vi "UV-VIS SetFastExtTriggerSD.vi"(3 "error in (no error)":errorcluster, 4 "mode":bool, 5 "Control in":refnum<class "CCD_camera.lvclass">) -> (0 "error out":errorcluster, 1 "DLL error code":u32, 2 "Control out":refnum<class "CCD_camera.lvclass">)   [LabVIEW 2018, in "CCD_camera.lvclass"]
doc: "This function will enable fast external triggering. When fast external triggering is enabled the system will NOT wait until a \"Keep Clean\" cycle has been completed before accepting the next trigger. This setting will only have an effect is the trigger mode has been set to External via <B>SetTriggerMode</B>.\n\n<B>Parameter:</B>\nmode - FALSE - Disabled\n TRUE - Enabled\n\n<B>Error code:</B>\nDRV_SUCCESS - Parameters accepted."
uses:
  CCD_camera.lvclass
  C:/Users/Sergey Denisov/Documents/REPS/TRANCON/Classes/Detector/Detector.lvclass
  Detector.lvclass/Detector.ctl
  Detector.lvclass
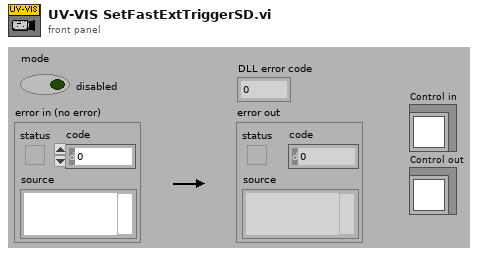
[diagram p1: front panel]
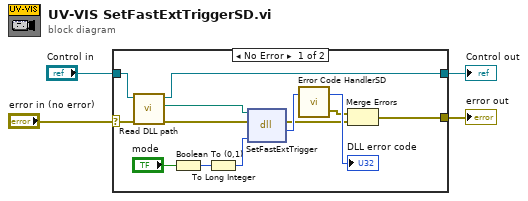
[diagram p0: block diagram]
diagram:
  n1 = case shown="No Error" "error in (no error)" {
    selector: "error in (no error)" -> [w11 w19]
    tunnel: [w6 w19] -> w3
    tunnel: [w5 w18] -> w2
    tunnel: "Control in" -> [w12 w18]
    frame No Error {
      n2 = call "Read DLL path.vi"("error in (no error)"=w11, "Detector in"=w12) -> ("error out"=w10:errorcluster, "DLL path"=w9:path, "Detector out"=w5:refnum<class "CCD_camera.lvclass">)  [unwired: 7 in]
      n3 = Boolean To (0,1)(Boolean="mode") -> (0, 1=w14:i16)
      n4 = To Long Integer(number=w14) -> (32bit integer=w13:i32)
      n5 = dll-call lib="S:/TRANCON/DLL/Atmcd32d.dll" fn="SetFastExtTrigger"(path in=w9, error in=w10, "mode"=w13) -> (error out=w8:errorcluster, "return type"=w17:u32)  [unwired: 2 in, 1 out]
      n6 = call "Error Code HandlerSD.vi"("DLL error code"=w17) -> ("error out"=w7:errorcluster, "dup DLL error code"=→"DLL error code":u32)  [unwired: 1 in]
      n7 = Merge Errors(w7, w8) -> (w6:errorcluster)
    }
    frame Error {
    }
  }
  "error out" <- w3
  "Control out" <- w2
